vi "LabJack_FGV_T4.vi"(6 "Operation(Read)":enum16{"Write", "Read"}(ring)=enum."Read", 8 "error in (no error)":errorcluster, 11 "Write data":i32) -> (0 "error out":errorcluster, 3 "Read data":i32)   [LabVIEW 2020]
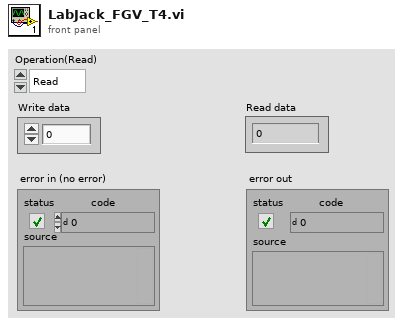
[diagram p1: front panel]
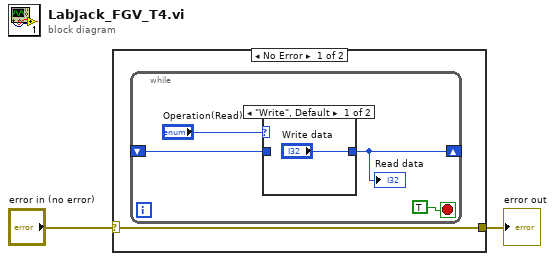
[diagram p0: block diagram]
diagram:
  n1 = case shown="No Error" "error in (no error)" {
    selector: "error in (no error)" -> [w3 w10]
    tunnel: [w3 w10] -> w1
    frame No Error {
      n2 = while {
        shift-right: [w5] -> _
        shift-left: _ -> [w4]
        stop <- TRUE stop-if-true
        n3 = case shown="\"Write\", Default" "Operation(Read)" {
          tunnel: ["Write data" w9] -> w5
          tunnel: w4 -> [_ w9]
          frame "Write", Default {
          }
          frame "Read" {
          }
        }
        "Read data" <- w5
      }
    }
    frame Error {
    }
  }
  "error out" <- w1
